vi "ST5520_CMD_2.vi"(8 "errin":errorcluster caption="entrée d'erreur (pas d'erreur)", 10 "VISA":string) -> (0 "errout":errorcluster caption="sortie d'erreur", 1 "DATA OUT FLT":dbl, 2 "DATA OUT STR":string, 3 "60s?":bool)   [LabVIEW 2020]
uses:
  VG/VG_progressBar.vi
  <instrlib>/HIOKI BT356X Series/HIOKI BT356X Series.lvlib
panel:
  in  "Arrêter":bool
  out "DATA LIVE":string
  # "DATA OUT"
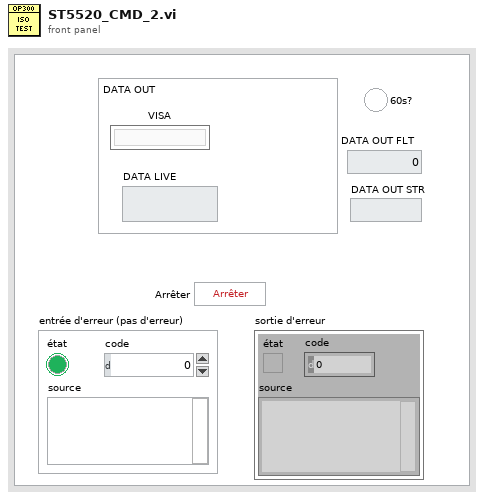
[diagram p1: front panel]
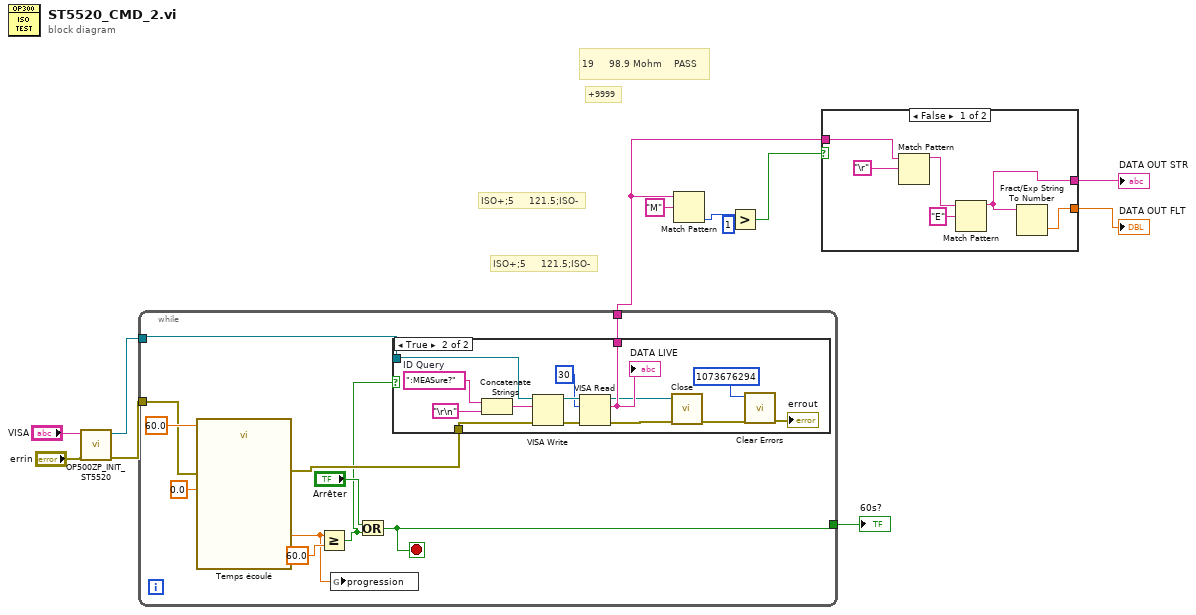
[diagram p0: block diagram]
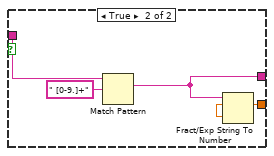
[diagram p2: hidden frame]
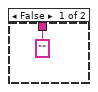
[diagram p3: hidden frame]
diagram:
  # "+9999"
  # "19     98.9 Mohm    PASS"
  # "ISO+;5     121.5;ISO-"
  # "ISO+;5     121.5;ISO-"
  n1 = call "OP500ZP_INIT_ST5520.vi"("errin"="errin", "VISA"="VISA") -> ("errout"=w10:errorcluster, "VISA"=w11:refnum<visa-resource-name>)  [unwired: 8 in]
  n2 = while {
    tunnel: w10 -> [w17]
    tunnel: w11 -> [w23]
    tunnel: [w19] -> w1
    tunnel: [w18] -> w12
    stop <- w18 stop-if-true
    n3 = call "Temps écoulé"("Time Target (s)"=60.0, "error in (no error)"=w17, "Set Start Time (s)"=0.0) -> ("Elapsed Time (s)"=w14:dbl, "error out"=w15:errorcluster)  [unwired: 9 in, 6 out]
    n4 = Greater Or Equal?(x=w14, y=60.0) -> (x >= y?=w13:bool)
    n5 = global write "VG_progressBar.vi" "progression"(w14) -> ()
    n6 = Or(x="Arrêter", y=w13) -> (x .or. y?=w18:bool)
    n7 = case shown="True" w13 {
      tunnel: w23 -> [_ w32]
      tunnel: ["" ("read buffer") w29] -> w19
      tunnel: w15 -> [_ w25]
      frame False {
      }
      frame True {
        w38 = ":MEASure?"  # ID Query
        n8 = Concatenate Strings(w38, "\r\n") -> (w34:string)
        n9 = VISA Write(VISA resource name=w32, write buffer=w34, error in (no error)=w25) -> (VISA resource name out=w37:refnum<visa-resource-name>, error out=w36:errorcluster)  [unwired: 1 out]
        n10 = VISA Read(VISA resource name=w37, byte count=u32 30 ("nombre d'octets"), error in (no error)=w36) -> (VISA resource name out=w26:refnum<visa-resource-name>, read buffer=w29:string, error out=w28:errorcluster)  [unwired: 1 out]
        "DATA LIVE" <- w29
        n11 = call <instrlib>:"Close.vi"("error in (no error)"=w28, "VISA resource name"=w26) -> ("error out"=w27:errorcluster)  [unwired: 9 in]
        n12 = call <vilib>:"Clear Errors.vi"("error in (no error)"=w27, "specific error code to clear (0: all)"=1073676294) -> ("error out"=→"errout":errorcluster)  [unwired: 4 in, 1 out]
      }
    }
  }
  "60s?" <- w12
  n13 = Match Pattern(string=w1, regular expression="M") -> (offset past match=w6:i32)  [unwired: 1 in, 3 out]
  n14 = Greater?(x=w6, y=1) -> (0:w4:bool)
  n15 = case shown="False" w4 {
    tunnel: w1 -> [w43 w47]
    tunnel: [w39 w45] -> w3
    tunnel: [w42 w46] -> w2
    frame False {
      n16 = Match Pattern(string=w43, regular expression="\r" ("expression régulière")) -> (before substring=w41:string)  [unwired: 1 in, 3 out]
      n17 = Match Pattern(string=w41, regular expression="E") -> (before substring=w39:string)  [unwired: 1 in, 3 out]
      n18 = Fract/Exp String To Number(string=w39) -> (number=w42:dbl)  [unwired: 3 in, 1 out]
    }
    frame True {
      n19 = Match Pattern(string=w47, regular expression=" [0-9.]+") -> (match substring=w45:string)  [unwired: 1 in, 3 out]
      n20 = Fract/Exp String To Number(string=w45) -> (number=w46:dbl)  [unwired: 3 in, 1 out]
    }
  }
  "DATA OUT STR" <- w3
  "DATA OUT FLT" <- w2
